vi "write_attributes.vi"(8 "error in (no error)":errorcluster, 10 "attributes":T1, 11 "FastICA in":refnum<class "FastICA.lvclass">) -> (0 "error out":errorcluster, 3 "FastICA out":refnum<class "FastICA.lvclass">)   [LabVIEW 2020, in "FastICA.lvclass"]
uses:
  FastICA.lvclass
  Controls/fast_ica_attributes.ctl
  FastICA.lvclass/FastICA.ctl
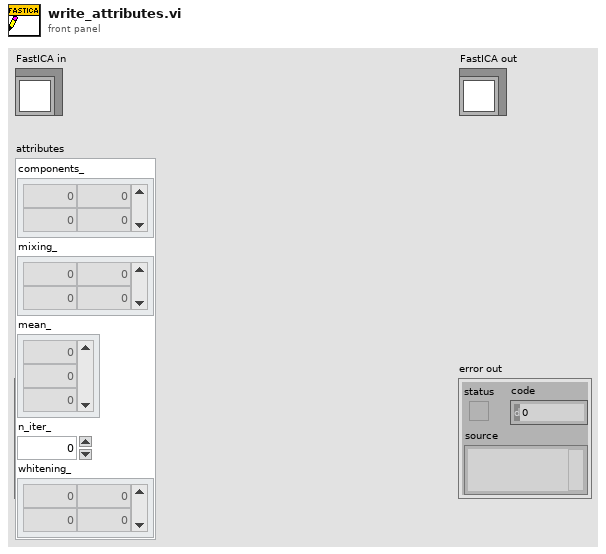
[diagram p1: front panel]
types:
  T1 = typedef "fast_ica_attributes.ctl" = cluster{"components_":dbl[][], "mixing_":dbl[][], "mean_":dbl[], "n_iter_":dbl, "whitening_":dbl[][]}
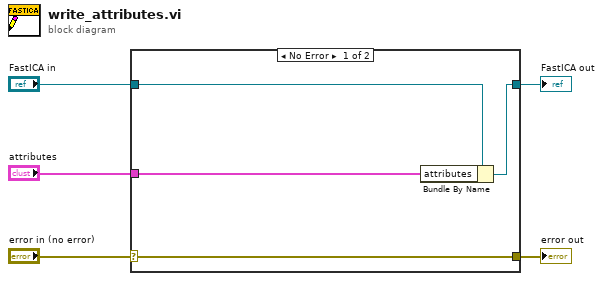
[diagram p0: block diagram]
diagram:
  n1 = case shown="No Error" "error in (no error)" {
    selector: "error in (no error)" -> [w9 w10]
    tunnel: [w9 w10] -> w4
    tunnel: [w7 w11] -> w2
    tunnel: "FastICA in" -> [w8 w11]
    tunnel: "attributes" -> [w6 _]
    frame No Error {
      n2 = Bundle By Name(cluster=w8, "attributes"=w6) -> (w7:refnum<class "FastICA.lvclass">)
    }
    frame Error {
    }
  }
  "error out" <- w4
  "FastICA out" <- w2
